vi "调用子界面.vi"   [LabVIEW 2018]
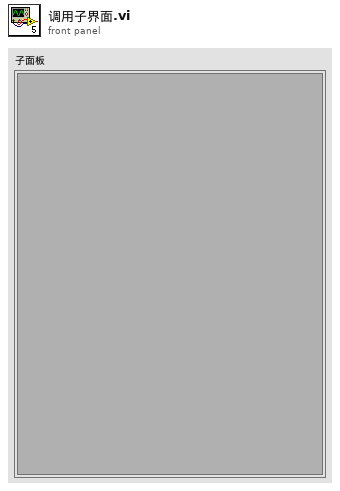
[diagram p1: front panel]
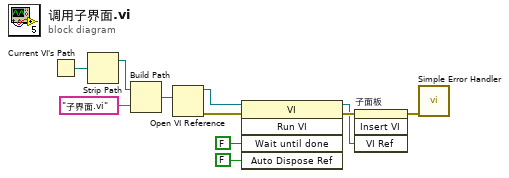
[diagram p0: block diagram]
diagram:
  n1 = Current VI's Path() -> (path=w11:path)
  n2 = Strip Path(path=w11) -> (stripped path=w10:path)  [unwired: 1 out]
  n3 = Build Path(base path=w10, name or relative path="子界面.vi" ("名称或相对路径")) -> (appended path=w8:path)
  n4 = Open VI Reference(vi path=w8) -> (vi reference=w7:refnum<vi>, error out=w2:errorcluster)  [unwired: 5 in]
  n5 = invoke class="VI" method="Run VI"(reference=w7, error in=w2, "Wait until done"=FALSE ("结束前等待"), "Auto Dispose Ref"=FALSE ("自动销毁引用")) -> (reference out=w3:refnum<vi>, error out=w4:errorcluster)  [unwired: 1 in, 3 out]
  n6 = invoke on="子面板" class="SubPnl" method="Insert VI"(error in=w4, "VI Ref"=w3) -> (error out=w1:errorcluster)  [unwired: 2 in, 3 out]
  n7 = call <vilib>:"Simple Error Handler.vi"("error in (no error)"=w1) -> ()  [unwired: 4 in, 5 out]
